vi "Tosca-Pupillometry Thread (EPL).vi"(0 "IPC":T1) -> (15 "error out":errorcluster)   [LabVIEW 2020]
uses:
  IPC VIs/Tosca-IPC.ctl
  Classes/Parameters/Parameters.lvclass
  Digital Input VIs/Tosca-DI Queue Data.ctl
  Digital Input VIs/Tosca-Input Event.ctl
  Digital Input VIs/Tosca-Input Criterion.ctl
  epl-vi-lib/Utility VIs/Type Defs/Logic State.ctl
  Typedefs/Tosca-Accumulator.ctl
  Typedefs/Tosca-State AODO.ctl
  Typedefs/Tosca-AO Runtime.ctl
  Typedefs/Tosca-DO Runtime.ctl
  epl-vi-lib/Signal Synthesis VIs/4th Generation/Classes/SignalManager/SignalManager.lvclass
  Typedefs/Tosca-Synapse Start Data.ctl
  IPC VIs/Tosca-Message.ctl
  IPC VIs/Tosca-Message Action.ctl
  Typedefs/Tosca-Thread Type.ctl
  Imaging VIs/Tosca-2P-Notifier Data.ctl
  Typedefs/Tosca-MATLAB Queue Data.ctl
  Visual Stim VIs/Tosca-Grating.ctl
  Visual Stim VIs/Tosca-Grating Type.ctl
  Typedefs/Tosca-File IO Notification.ctl
  epl-vi-lib/TCP VIs/TCP Params.ctl
  epl-vi-lib/TCP VIs/TCP Write.vi
  Sub VIs/Tosca-Globals.vi
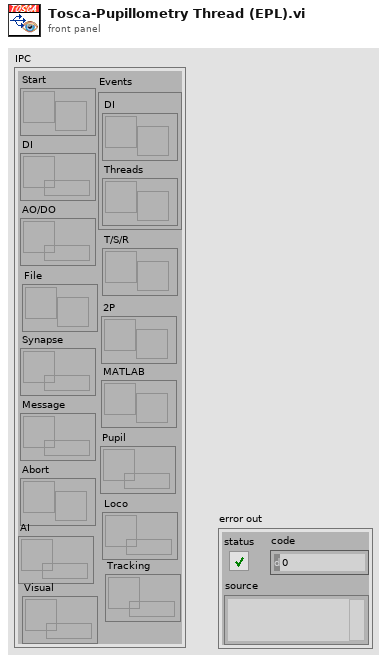
[diagram p1: front panel]
types:
  T1 = typedef "Tosca-IPC.ctl" = cluster{"Start":refnum<notifier>, "DI":refnum<queue>, "AO/DO":refnum<queue>, "Synapse":refnum<queue>, "Message":refnum<queue>, "Abort":refnum<notifier>, "Events":cluster{"DI":refnum<user-event>, "Threads ":refnum<user-event>}, "T/S/R":refnum<notifier>, "2P":refnum<notifier>, "MATLAB":refnum<notifier>, "Pupil":refnum<queue>, "Loco":refnum<queue>, "AI":refnum<queue>, "Tracking":refnum<queue>, "Visual":refnum<queue>, "File":refnum<notifier>}
  T2 = enum16{"big-endian, network order", "native, host order", "little-endian"}
  T3 = typedef "TCP Params.ctl" = cluster{"IP Address":string, "Port":i32}
  T4 = typedef "Tosca-Thread Type.ctl" = enum16{"None", "AODO", "Masker", "ET", "Imaging", "Pupil", "AI", "DI", "Camera", "TTL out", "Loco", "Visual"}
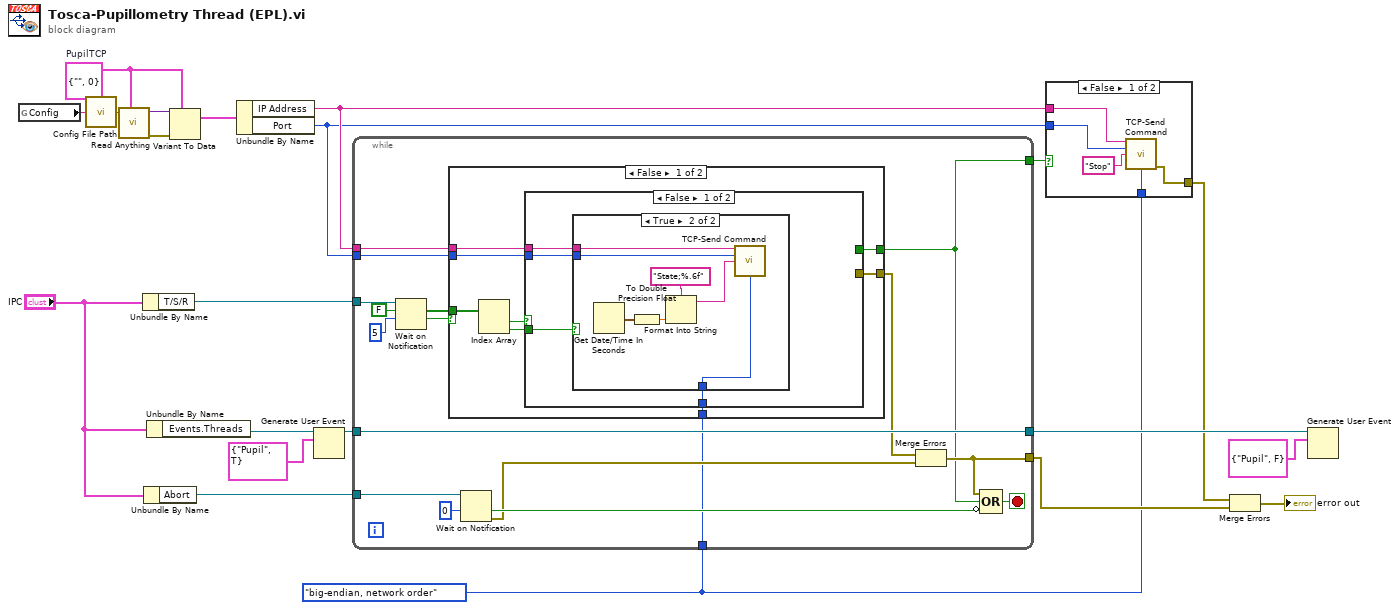
[diagram p0: block diagram]
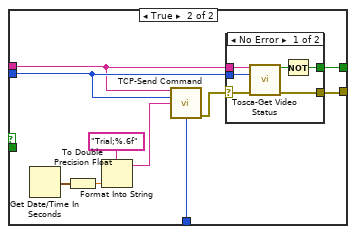
[diagram p3: hidden frame]
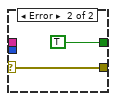
[diagram p4: hidden frame]
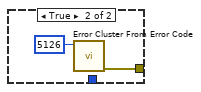
[diagram p6: hidden frame]
diagram:
  w1 = T2."big-endian, network order" ("byte order")
  w12 = T3 {"IP Address"="", "Port"=0}  # PupilTCP
  n1 = global read "Tosca-Globals.vi" "Config"() -> (w2:string)
  n2 = call "Config File Path.vi"("AppName"=w2) -> ("Default config file name"=w11:path)
  n3 = call "Read Anything.vi"("Type of Anything"=w12, "Path (dialog)"=w11) -> ("Error Out"=w14:errorcluster, "Anything"=w13:variant)  [unwired: 7 in, 1 out]
  n4 = Unbundle By Name("IPC") -> ("T/S/R"=w3:refnum<notifier>)
  n5 = Unbundle By Name("IPC") -> ("Abort"=w16:refnum<notifier>)
  n6 = Unbundle By Name("IPC") -> ("Events.Threads"=w21:refnum<user-event>)
  n7 = Variant To Data(error in=w14, type=w12, Variant=w13) -> (data=w15:T3)  [unwired: 1 out]
  n8 = Unbundle By Name(w15) -> ("IP Address"=w6:string, "Port"=w5:i32)
  n9 = Generate User Event(user event=w21, event data cluster=cluster{"ID":T4, "Running":bool} {"ID"=enum."Pupil", "Running"=TRUE} ("event data")) -> (user event out=w19:refnum<user-event>)  [unwired: 2 in, 1 out]
  n10 = while {
    tunnel: w19 -> [w38]
    tunnel: [w38] -> w18
    tunnel: w16 -> [w35]
    tunnel: w6 -> [w24]
    tunnel: w5 -> [w25]
    tunnel: [w31] -> w9
    tunnel: [w32] -> w8
    tunnel: w3 -> [w28]
    tunnel: w1 -> [w22]
    stop <- w34 stop-if-true
    n11 = Wait on Notification(notifier=w28, ignore previous (F)=FALSE, timeout in ms (-1)=5) -> (notification=w26:bool[], timed out?=w27:bool)  [unwired: 1 in, 2 out]
    n12 = case shown="False" w27 {
      tunnel: w26 -> [w45 _]
      tunnel: w24 -> [w44 _]
      tunnel: w25 -> [w43 _]
      tunnel: [w42 _] -> w23
      tunnel: [w41 _] -> w31
      tunnel: w22 -> [w39 _]
      frame False {
        n13 = Index Array(array=w45) -> (element #1=w46:bool, element #2=w40:bool)  [unwired: 2 in]
        n14 = case shown="False" w46 {
          tunnel: w44 -> [w49 w61]
          tunnel: w43 -> [w48 w62]
          tunnel: [_ w60] -> w42
          tunnel: [_ w59] -> w41
          tunnel: w40 -> [w50 _]
          tunnel: w39 -> [w47 w58]
          frame False {
            n15 = case shown="True" w50 {
              tunnel: w49 -> [_ w52]
              tunnel: w48 -> [_ w53]
              tunnel: w47 -> [_ w51]
              frame False {
              }
              frame True {
                n16 = Get Date/Time In Seconds() -> (seconds since 1Jan1904=w55:timestamp)
                n17 = To Double Precision Float(number=w55) -> (double precision float=w54:dbl)
                n18 = Format Into String(format string="State;%.6f", w54) -> (resulting string=w56:string)  [unwired: 2 in, 1 out]
                n19 = call "TCP-Send Command.vi"("PXI Address"=w52, "Port"=w53, "Command"=w56, "byte order"=w51) -> ()  [unwired: 11 in, 1 out]
              }
            }
          }
          frame True {
            n20 = Get Date/Time In Seconds() -> (seconds since 1Jan1904=w65:timestamp)
            n21 = To Double Precision Float(number=w65) -> (double precision float=w64:dbl)
            n22 = Format Into String(format string="Trial;%.6f", w64) -> (resulting string=w66:string)  [unwired: 2 in, 1 out]
            n23 = call "TCP-Send Command.vi"("PXI Address"=w61, "Port"=w62, "Command"=w66, "byte order"=w58) -> ("error out"=w63:errorcluster)  [unwired: 11 in]
            n24 = case shown="No Error" w63 {
              selector: w63 -> [w73 w75]
              tunnel: w62 -> [w72 _]
              tunnel: w61 -> [w71 _]
              tunnel: [w70 w75] -> w60
              tunnel: [w68 TRUE ("Recording")] -> w59
              frame No Error {
                n25 = call "Tosca-Get Video Status.vi"("IP Address"=w71, "Port"=w72, "error in (no error)"=w73) -> ("Recording"=w69:bool, "error out"=w70:errorcluster)  [unwired: 11 in]
                n26 = Not(x=w69) -> (.not. x?=w68:bool)
              }
              frame Error {
              }
            }
          }
        }
      }
      frame True {
      }
    }
    n27 = Wait on Notification(notifier=w35, timeout in ms (-1)=0) -> (timed out?=w37:bool, error out=w33:errorcluster)  [unwired: 2 in, 2 out]
    n28 = Merge Errors(w23, w33) -> (w32:errorcluster)
    n29 = Compound Arithmetic op=OR(w32, w31, invert w37) -> (w34:bool)
  }
  n30 = case shown="False" w9 {
    tunnel: [w77 w81] -> w7
    tunnel: w6 -> [w79 _]
    tunnel: w5 -> [w78 _]
    tunnel: w1 -> [w76 _]
    frame False {
      n31 = call "TCP-Send Command.vi"("PXI Address"=w79, "Port"=w78, "Command"="Stop", "byte order"=w76) -> ("error out"=w77:errorcluster)  [unwired: 11 in]
    }
    frame True {
      n32 = call <vilib>:"Error Cluster From Error Code.vi"("error code (0)"=5126) -> ("error out"=w81:errorcluster)  [unwired: 8 in]
    }
  }
  n33 = Merge Errors(w7, w8) -> (→"error out":errorcluster)
  n34 = Generate User Event(user event=w18, event data cluster=cluster{"ID":T4, "Running":bool} {"ID"=enum."Pupil", "Running"=FALSE} ("event data")) -> ()  [unwired: 2 in, 2 out]
